vi "ChoseTarget.vi"(0 "center3":cluster{dbl, dbl}, 4 "center2":cluster{dbl, dbl}, 6 "center1":cluster{dbl, dbl}, 9 "distance3":dbl, 10 "distance2":dbl, 11 "distance1":dbl) -> (2 "ChosenCenter":cluster{dbl, dbl}, 3 "ChosenDistance":dbl)   [LabVIEW 2015]
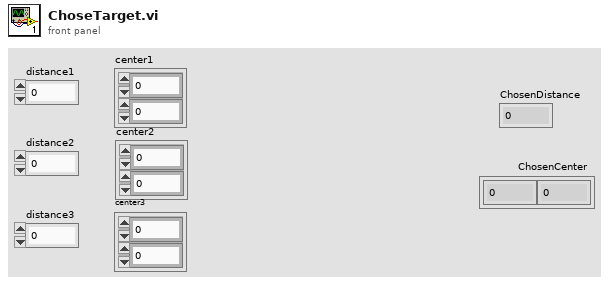
[diagram p1: front panel]
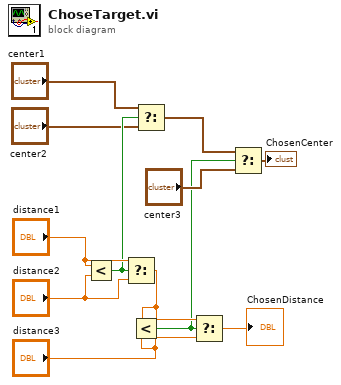
[diagram p0: block diagram]
diagram:
  n1 = Less?(x="distance1", y="distance2") -> (x < y?=w7:bool)
  n2 = Select(t="distance1", s=w7, f="distance2") -> (s? t:f=w10:dbl)
  n3 = Less?(x=w10, y="distance3") -> (x < y?=w2:bool)
  n4 = Select(t="center1", s=w7, f="center2") -> (s? t:f=w3:cluster{dbl, dbl})
  n5 = Select(t=w10, s=w2, f="distance3") -> (s? t:f=→"ChosenDistance":dbl)
  n6 = Select(t=w3, s=w2, f="center3") -> (s? t:f=→"ChosenCenter":cluster{dbl, dbl})
